vi "Requests.vi"(8 "error in (no error)":errorcluster, 9 "write enable":bool=TRUE, 11 "ICPCON ET-7016 in":refnum<class "ICPCON ET-7016.lvclass">) -> (0 "error out":errorcluster, 3 "ICPCON ET-7016 out":refnum<class "ICPCON ET-7016.lvclass">)   [LabVIEW 2019, in "ICPCON ET-7016.lvclass"]
uses:
  ICPCON ET-7016.lvclass
  D:/my_projects/projects/Algorithms/Labview/19/Modbus/MB_TCP2/MB_TCP.lvclass
  MB_TCP.lvclass/MB_TCP.ctl
  NI_modbus_upd/Ctl/Unit_ID.ctl
  NI_modbus_upd/TCP/TCP.lvclass/TCP.ctl
  NI_modbus_upd/Master Function Definition/Responses/Read Input Registers Response.vi
  NI_modbus_upd/Master network read write.vi
  NI_modbus_upd/Master Function Definition/Requests/Read Input Registers Request.vi
  NI_modbus_upd/Master Function Definition/Responses/Read Coils Response.vi
  NI_modbus_upd/Master Function Definition/Requests/Read Coils Request.vi
  NI_modbus_upd/Master Function Definition/Responses/Read Discrete Inputs Response.vi
  NI_modbus_upd/Master Function Definition/Requests/Read Discrete Inputs Request.vi
  NI_modbus_upd/Utility/Bytes to U16s1.vi
  NI_modbus_upd/Function code mismatch error1.vi
  NI_modbus_upd/Error Generator1.vi
  NI_modbus_upd/Read ADU Packet Master.vi
  NI_modbus_upd/Write ADU Packet Master.vi
  NI_modbus_upd/Modbus Data Unit (PDU)/Construct PDU1.vi
  NI_modbus_upd/Utility/Bytes to Bits1.vi
  NI_modbus_upd/Modbus Data Unit (PDU)/Unflatten to PDU1.vi
  NI_modbus_upd/TCP/Protocol Read.vi
  NI_modbus_upd/TCP/Protocol Write.vi
  <vilib>/Utility/error.llb/Clear Errors.vi
  NI_modbus_upd/Modbus Data Unit (PDU)/Deconstruct PDU1.vi
  NI_modbus_upd/TCP/TCP.lvclass
  ICPCON Registers/ICPCON Registers.lvlib
  MB_TCP.lvclass
  NI_modbus_upd/NI_modbus_upd.lvlib
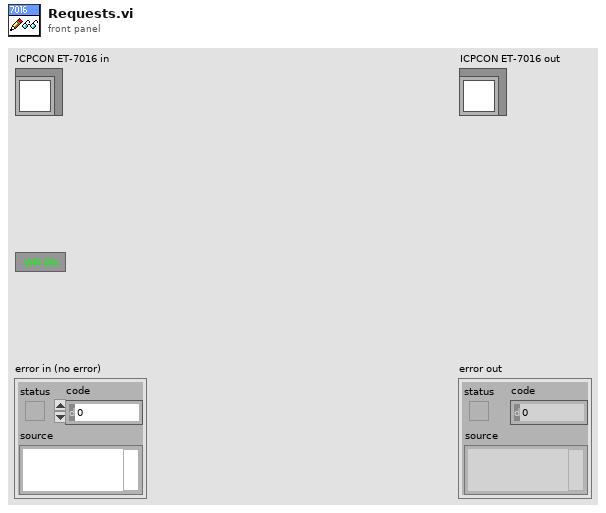
[diagram p1: front panel]
types:
  T1 = typedef "NI_modbus_upd.lvlib/Unit_ID.ctl" = cluster{"Protocol ID":u16, "Unit ID":u8}
  T2 = typedef "ICPCON Registers.lvlib/ICPCON Data.ctl" = cluster{"UTF":refnum<data-value>, "DI":refnum<data-value>, "DW":refnum<data-value>, "DO":refnum<data-value>, "IR":refnum<data-value>, "WR":refnum<data-value>, "OR":refnum<data-value>, "modified":refnum<data-value>}
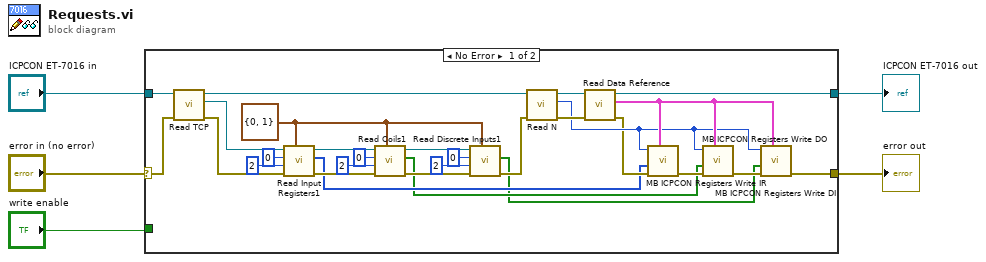
[diagram p0: block diagram]
diagram:
  n1 = case shown="No Error" "error in (no error)" {
    selector: "error in (no error)" -> [w26 w36]
    tunnel: [w29 w36] -> w3
    tunnel: [w24 w35] -> w4
    tunnel: "ICPCON ET-7016 in" -> [w27 w35]
    tunnel: "write enable" -> [_ _]
    frame No Error {
      w13 = T1 {"Protocol ID"=0, "Unit ID"=1} ("Unit_ID")
      n2 = call "Read TCP.vi"("error in (no error)"=w26, "MB_TCP in"=w27) -> ("error out"=w22:errorcluster, "TCP"=w23:refnum<class "TCP.lvclass">, "MB_TCP out"=w25:refnum<class "ICPCON ET-7016.lvclass">)  [unwired: 7 in]
      n3 = call "Read Input Registers1.vi"("Unit_ID"=w13, "error in (no error)"=w22, "number of input registers"=u16 2, "starting address"=u16 0, "Modbus master in"=w23) -> ("error out"=w18:errorcluster, "register values"=w8:u16[], "Modbus master out"=w19:refnum<class "TCP.lvclass">)  [unwired: 4 in]
      n4 = call "Read Coils1.vi"("Unit_ID"=w13, "error in (no error)"=w18, "number of coils"=u16 2, "starting address"=u16 0, "Modbus master in"=w19) -> ("error out"=w11:errorcluster, "coil values"=w7:bool[], "Modbus master out"=w12:refnum<class "TCP.lvclass">)  [unwired: 4 in]
      n5 = call "Read Discrete Inputs1.vi"("Unit_ID"=w13, "error in (no error)"=w11, "number of discrete inputs"=u16 2 ("number of coils"), "starting address"=u16 0, "Modbus master in"=w12) -> ("error out"=w10:errorcluster, "discrete input values"=w6:bool[])  [unwired: 4 in, 1 out]
      n6 = call "Read N.vi"("error in (no error)"=w10, "MB_TCP in"=w25) -> ("error out"=w34:errorcluster, "N"=w28:i32, "MB_TCP out"=w33:refnum<class "ICPCON ET-7016.lvclass">)  [unwired: 7 in]
      n7 = call "Read Data Reference.vi"("error in (no error)"=w34, "MB_TCP in"=w33) -> ("error out"=w9:errorcluster, "Data"=w30:T2, "MB_TCP out"=w24:refnum<class "ICPCON ET-7016.lvclass">)  [unwired: 7 in]
      n8 = call "MB ICPCON Registers Write IR.vi"("Data Reference"=w30, "error in (no error)"=w9, "Words In"=w8, "N"=w28) -> ("error out"=w32:errorcluster)  [unwired: 7 in]
      n9 = call "MB ICPCON Registers Write DO.vi"("Data Reference"=w30, "error in (no error)"=w32, "Bits In"=w7, "N"=w28) -> ("error out"=w31:errorcluster)  [unwired: 7 in]
      n10 = call "MB ICPCON Registers Write DI.vi"("Data Reference"=w30, "error in (no error)"=w31, "Bits In"=w6, "N"=w28) -> ("error out"=w29:errorcluster)  [unwired: 7 in]
    }
    frame Error {
    }
  }
  "error out" <- w3
  "ICPCON ET-7016 out" <- w4
